vi "AH_GetMSG.vi"(7 "byte count":u32=1024, 8 "error in (no error)":errorcluster, 9 "Halt For RQS":bool, 10 "Data Cluster In":T1 {"GUI Data Cluster"."SBR" format="%08b"}, 11 "Config Cluster In":T3={"General"={"Config.ini"=path "", "Default Logging Path"=path ""}, "Hardware"={"AHC VISA COM"="", "Measure Rate (1/s)"=0, "Global T VAR"="", "Global B VAR"="", "Average"=4, "Bias"=0, "Cable"={"Length"=0.0, "Resistance"=0.0, "Inductance"=0.0, "Capacitance"=0.0}, "Tracking"=0, "Voltage"=0.0}, "Operation"={"Operation Mode"=enum."Logging", "Status"="", "NewLog?"=FALSE}}) -> (0 "error IO":errorcluster, 1 "read buffer":string, 2 "Data Cluster Out":T1 {"GUI Data Cluster"."SBR" format="%08b"}, 3 "Configuration Cluster Out":T3={"General"={"Config.ini"=path "", "Default Logging Path"=path ""}, "Hardware"={"AHC VISA COM"="", "Measure Rate (1/s)"=0, "Global T VAR"="", "Global B VAR"="", "Average"=4, "Bias"=0, "Cable"={"Length"=0.0, "Resistance"=0.0, "Inductance"=0.0, "Capacitance"=0.0}, "Tracking"=0, "Voltage"=0.0}, "Operation"={"Operation Mode"=enum."Idle-Off", "Status"="", "NewLog?"=FALSE}}, 4 "MSG Res":bool, 6 "SRQ Timed Out":bool)   [LabVIEW 2021]
uses:
  Config_Cluster.ctl
  Mode_Enum.ctl
  Data_Cluster.ctl
  Measurement_Cluster.ctl
  Status_Byte.ctl
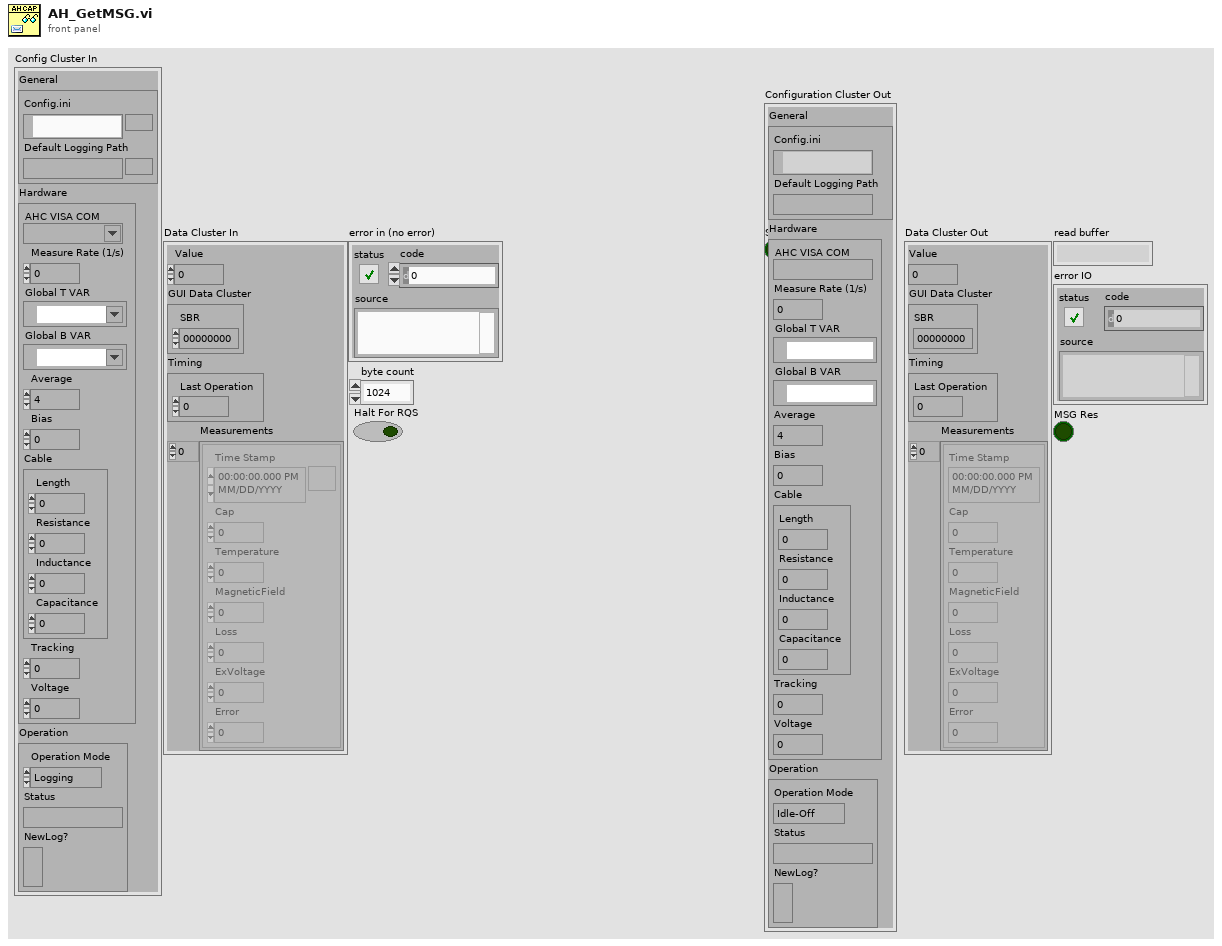
[diagram p1: front panel]
types:
  T1 = typedef "Data_Cluster.ctl" = cluster{"Value":dbl, "GUI Data Cluster":cluster{"SBR":u16}, "Timing":cluster{"Last Operation":dbl}, "Measurements":T2[]}
  T2 = typedef "Measurement_Cluster.ctl" = cluster{"Time Stamp":timestamp, "Cap":dbl, "Temperature":dbl, "MagneticField":dbl, "Loss":dbl, "ExVoltage":dbl, "Error":dbl}
  T3 = typedef "Config_Cluster.ctl" = cluster{"General":cluster{"Config.ini":path, "Default Logging Path":path}, "Hardware":cluster{"AHC VISA COM":refnum<visa-resource-name>, "Measure Rate (1/s)":i32, "Global T VAR":refnum<k21>, "Global B VAR":refnum<k21>, "Average":u8, "Bias":u8, "Cable":cluster{"Length":dbl, "Resistance":dbl, "Inductance":dbl, "Capacitance":dbl}, "Tracking":u8, "Voltage":dbl}, "Operation":cluster{"Operation Mode":T4, "Status":string, "NewLog?":bool}}
  T4 = typedef "Mode_Enum.ctl" = enum16{"Logging", "Idle-Off", "Idle"}
  T5 = typedef "Status_Byte.ctl" = u16
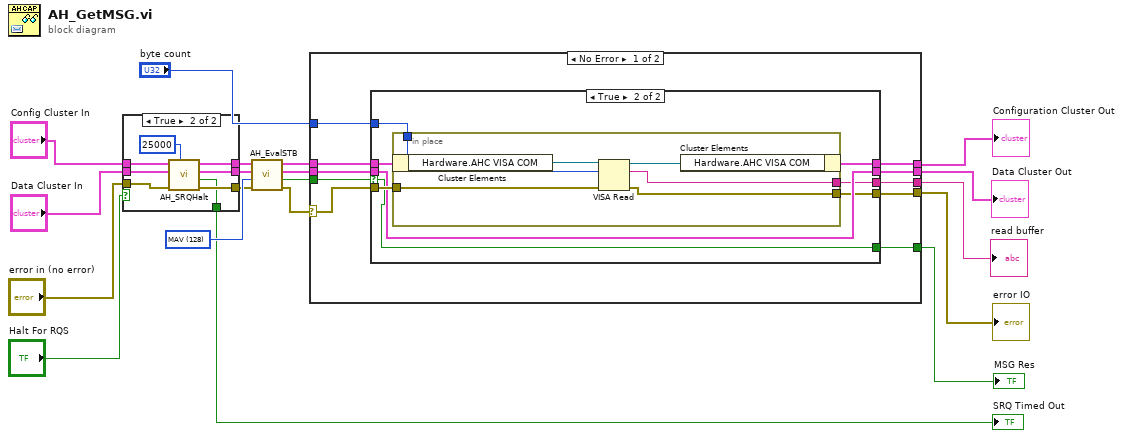
[diagram p0: block diagram]
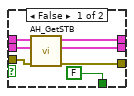
[diagram p2: hidden frame]
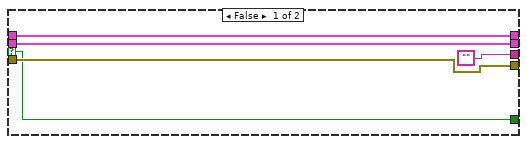
[diagram p3: hidden frame]
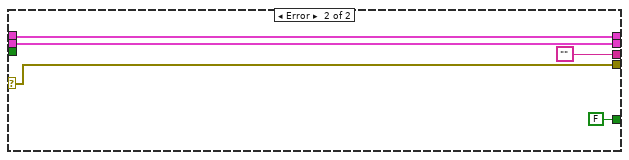
[diagram p4: hidden frame]
diagram:
  w14 = T5 128 items=["ONR"=1, "CME"=2, "URQ"=4, "PON"=8, "RDY"=16, "EXE"=32, "RQS"=64, "MAV"=128] ("Status Byte")
  n1 = case shown="True" "Halt For RQS" {
    tunnel: "Config Cluster In" -> [w26 w34]
    tunnel: "Data Cluster In" -> [w25 w33]
    tunnel: "error in (no error)" -> [w24 w28]
    tunnel: [w23 w31] -> w16
    tunnel: [w22 w30] -> w15
    tunnel: [w21 w29] -> w13
    tunnel: [FALSE ("SRQ Timed Out") w27] -> w6
    frame False {
      n2 = call "AH_GetSTB.vi"("error in (no error)"=w24, "Data Cluster In"=w25, "Config Cluster In"=w26) -> ("error out"=w21:errorcluster, "Data Cluster Out"=w22:T1, "Configuration Cluster Out"=w23:T3)  [unwired: 6 in]
    }
    frame True {
      n3 = call "AH_SRQHalt.vi"("timeout"=u32 25000, "error in (no error)"=w28, "Data Cluster In"=w33, "Config Cluster In"=w34) -> ("error out"=w29:errorcluster, "SRQ Timed Out"=w27:bool, "Data Cluster Out"=w30:T1, "Configuration Cluster Out"=w31:T3)  [unwired: 4 in]
    }
  }
  "SRQ Timed Out" <- w6
  n4 = call "AH_EvalSTB.vi"("error in (no error)"=w13, "Status Byte"=w14, "Data Cluster In"=w15, "Config Cluster In"=w16) -> ("error out"=w8:errorcluster, "Result"=w12:bool, "Data Cluster Out"=w11:T1, "Configuration Cluster Out"=w10:T3)  [unwired: 3 in, 1 out]
  n5 = case shown="No Error" w8 {
    selector: w8 -> [w40 w66]
    tunnel: w12 -> [w44 _]
    tunnel: w11 -> [w43 w67]
    tunnel: w10 -> [w42 w68]
    tunnel: "byte count" -> [w41 _]
    tunnel: [w39 w68] -> w5
    tunnel: [w38 w67] -> w4
    tunnel: [w36 w66] -> w2
    tunnel: [w37 ""] -> w3
    tunnel: [w35 FALSE] -> w1
    frame No Error {
      n6 = case shown="True" w44 {
        selector: w44 -> [w45 w50]
        tunnel: w40 -> [w46 w55]
        tunnel: w43 -> [w48 w53]
        tunnel: w42 -> [w49 w57]
        tunnel: w41 -> [_ w56]
        tunnel: [w49 w54] -> w39
        tunnel: [w48 w53] -> w38
        tunnel: ["" w52] -> w37
        tunnel: [w46 w51] -> w36
        tunnel: [w45 w50] -> w35
        frame False {
        }
        frame True {
          n7 = in-place {
            in-place-border: w56 -> [w61]
            in-place-border: w55 -> [w60]
            in-place-border: [w59] -> w52
            in-place-border: [w58] -> w51
            n8 = in-place-cluster #1(w57) -> ("Hardware.AHC VISA COM"=w63:refnum<visa-resource-name>)
            n9 = VISA Read(VISA resource name=w63, byte count=w61, error in (no error)=w60) -> (VISA resource name out=w62:refnum<visa-resource-name>, read buffer=w59:string, error out=w58:errorcluster)  [unwired: 1 out]
            n10 = in-place-cluster #1("Hardware.AHC VISA COM"=w62) -> (w54:T3)
          }
        }
      }
    }
    frame Error {
    }
  }
  "Configuration Cluster Out" <- w5
  "Data Cluster Out" <- w4
  "read buffer" <- w3
  "error IO" <- w2
  "MSG Res" <- w1
